vi "MICSD ZL7010X ADC.vi"(0 "VISA Resource Name":refnum<visa-resource-name>, 1 "Execute on Remote?(F)":bool, 5 "ADC Select":u8, 11 "error in (no error)":errorcluster) -> (4 "dup VISA Resource Name":refnum<visa-resource-name>, 6 "ADC Reading":u8, 15 "error out":errorcluster)   [LabVIEW 2010]
uses:
  <vilib>/Instr/_visa.llb/VISA Configure Serial Port (Instr).vi
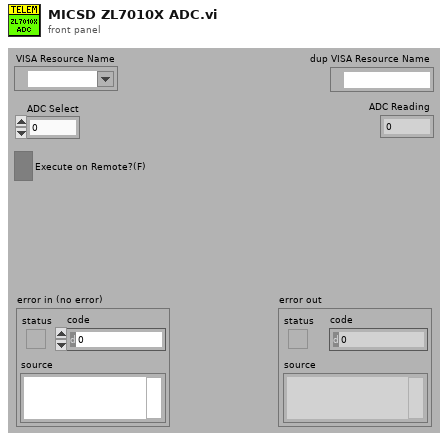
[diagram p1: front panel]
types:
  T1 = cluster{"Command Token":u8, "Length":u16, "Pack Data":u8[]}
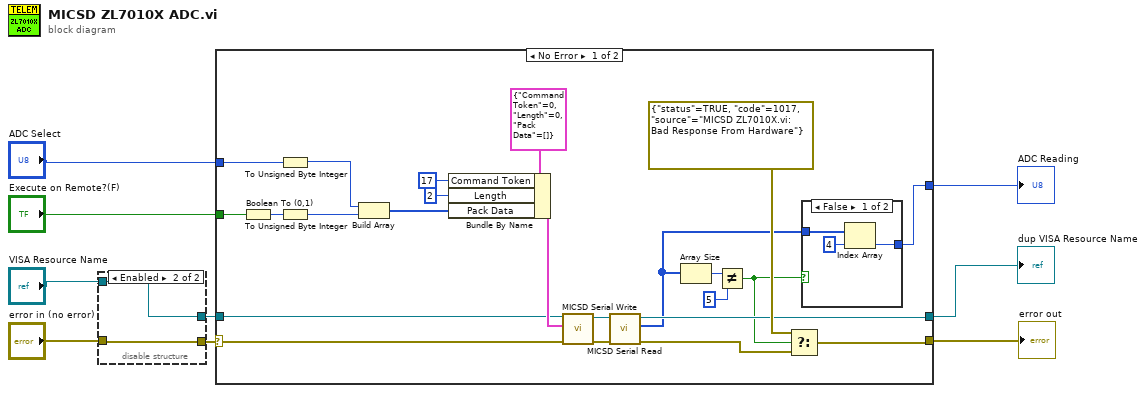
[diagram p0: block diagram]
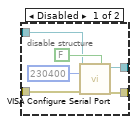
[diagram p2: hidden frame]
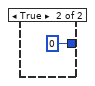
[diagram p3: hidden frame]
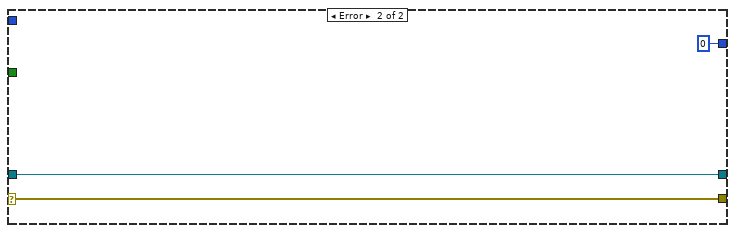
[diagram p4: hidden frame]
diagram:
  n1 = disable-structure shown="Enabled" {
    disable-tunnel: [w13 w16] -> w9
    disable-tunnel: [w12 w17] -> w8
    disable-tunnel: "VISA Resource Name" -> [w11 w17]
    disable-tunnel: "error in (no error)" -> [w10 w16]
    frame Disabled {
      n2 = call-poly "VISA Configure Serial Port"("VISA resource name"=w11, "Enable Termination\nChar (T)"=FALSE ("Enable Termination\nChar (T)"), "baud rate (9600)"=u32 230400, "error in (no error)"=w10) -> ("VISA resource name out"=w12:refnum<visa-resource-name>, "error out"=w13:errorcluster)  [unwired: 10 in]
    }
    frame Enabled {
    }
  }
  n3 = case shown="No Error" w9 {
    selector: w9 -> [w35 w46]
    tunnel: w8 -> [w36 w47]
    tunnel: "ADC Select" -> [w27 _]
    tunnel: "Execute on Remote?(F)" -> [w34 _]
    tunnel: [w21 w46] -> w4
    tunnel: [w22 w47] -> w5
    tunnel: [w18 u8 0 ("Source")] -> w1
    frame No Error {
      n4 = Boolean To (0,1)(Boolean=w34) -> (0, 1=w33:i16)
      n5 = To Unsigned Byte Integer(number=w27) -> (unsigned 8bit integer=w32:u8)
      n6 = To Unsigned Byte Integer(number=w33) -> (unsigned 8bit integer=w31:u8)
      n7 = Build Array(w32, w31) -> (w30:u8[])
      n8 = Bundle By Name(cluster=T1 {"Command Token"=0, "Length"=0, "Pack Data"=[]} ("Write Data"), "Command Token"=u8 17, "Length"=u16 2, "Pack Data"=w30) -> (w40:T1)
      n9 = call "MICSD Serial Write.vi"("error in (no error)"=w35, "Write Data"=w40, "VISA Resource Name"=w36) -> ("error out"=w28:errorcluster, "DUP Visa Resource Name"=w29:refnum<visa-resource-name>)  [unwired: 7 in]
      n10 = call "MICSD Serial Read.vi"("error in (no error)"=w28, "VISA Resource Name"=w29) -> ("error out"=w23:errorcluster, "Read Data"=w20:u8[], "DUP Visa Resource Name"=w22:refnum<visa-resource-name>)  [unwired: 7 in]
      n11 = Array Size(array=w20) -> (size(s)=w25:i32)
      n12 = Not Equal?(x=w25, y=5) -> (x != y?=w19:bool)
      n13 = Select(t=errorcluster {"status"=TRUE, "code"=1017, "source"="MICSD ZL7010X.vi:  Bad Response From Hardware"} ("error IO"), s=w19, f=w23) -> (s? t:f=w21:errorcluster)
      n14 = case shown="False" w19 {
        tunnel: w20 -> [w42 _]
        tunnel: [w41 u8 0 ("Source")] -> w18
        frame False {
          n15 = Index Array(array=w42, index=4) -> (element=w41:u8)
        }
        frame True {
        }
      }
    }
    frame Error {
    }
  }
  "dup VISA Resource Name" <- w5
  "error out" <- w4
  "ADC Reading" <- w1
